vi "ReadTrace.vi"(8 "error in (no error)":errorcluster, 11 "SpecA_ESA in":refnum<class "SpecA_ESA.lvclass">) -> (0 "error out":errorcluster, 2 "Trace Waveform":T1(graph), 3 "SpecA_ESA out":refnum<class "SpecA_ESA.lvclass">)   [LabVIEW 2014, in "SpecA_ESA.lvclass"]
uses:
  SpecA_ESA.lvclass
  SpecA_ESA.lvclass/SpecA_ESA.ctl
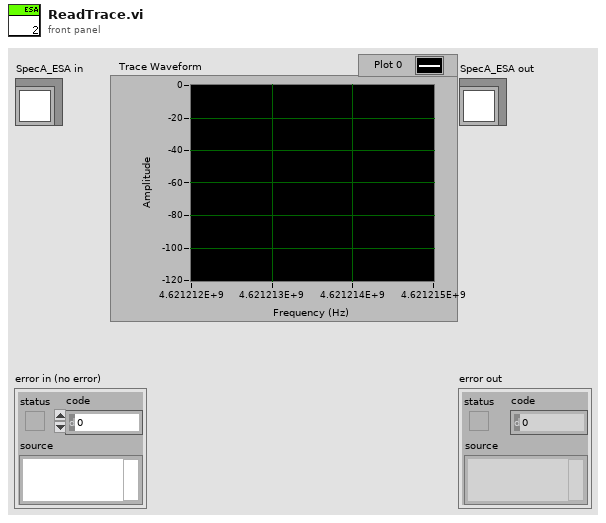
[diagram p1: front panel]
types:
  T1 = cluster{"Initial X":dbl, "X Increment":dbl, "Trace Array":dbl[]}
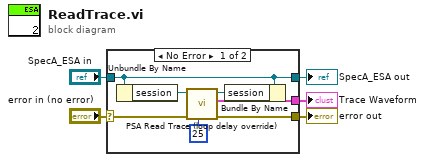
[diagram p0: block diagram]
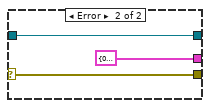
[diagram p2: hidden frame]
diagram:
  n1 = case shown="No Error" "error in (no error)" {
    selector: "error in (no error)" -> [w12 w13]
    tunnel: [w7 T1 {"Initial X"=0.0, "X Increment"=0.0, "Trace Array"=[]} ("Trace Waveform")] -> w4
    tunnel: [w11 w13] -> w3
    tunnel: "SpecA_ESA in" -> [w8 w14]
    tunnel: [w8 w14] -> w1
    frame No Error {
      n2 = Unbundle By Name(w8) -> ("session"=w10:refnum<visa-resource-name>)
      n3 = call "PSA Read Trace (loop delay override).vi"("loop delay (ms)"=u32 25, "error in (no error)"=w12, "VISA resource name"=w10) -> ("error out"=w11:errorcluster, "Trace Waveform"=w7:T1, "VISA resource name out"=w9:refnum<visa-resource-name>)  [unwired: 6 in]
      n4 = Bundle By Name(cluster=w8, "session"=w9) -> ()  [unwired: 1 out]
    }
    frame Error {
    }
  }
  "error out" <- w3
  "SpecA_ESA out" <- w1
  "Trace Waveform" <- w4
